vi "StringToAryy.vi"(11 "string":string) -> (3 "数组":string[](array[string]))   [LabVIEW 2018]
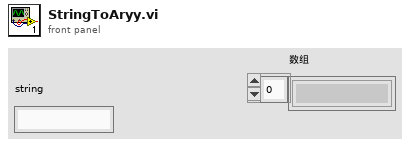
[diagram p1: front panel]
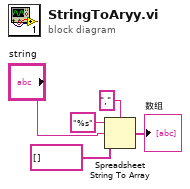
[diagram p0: block diagram]
diagram:
  n1 = Spreadsheet String To Array(delimiter (Tab)="," ("分隔符(Tab)"), format string="%s" ("格式字符串"), spreadsheet string="string", array type (2D Dbl)=string[] []) -> (array=→"数组":string[])
